vi "Initialize Sourcemeter (Pratap).vi"(5 "Source Value":dbl, 7 "Compliance Limit":dbl, 8 "error in (no error)":errorcluster, 9 "Reset (True)":bool, 10 "Source Function":enum32{"Current", "Voltage"}(ring), 11 "VISA Refnum in":refnum<visa-resource-name>) -> (0 "error out":errorcluster, 2 "Node Out":string, 3 "VISA Refnum out":refnum<visa-resource-name>)   [LabVIEW 2025, in "MySMU.lvlib"]
uses:
  MySMU.lvlib
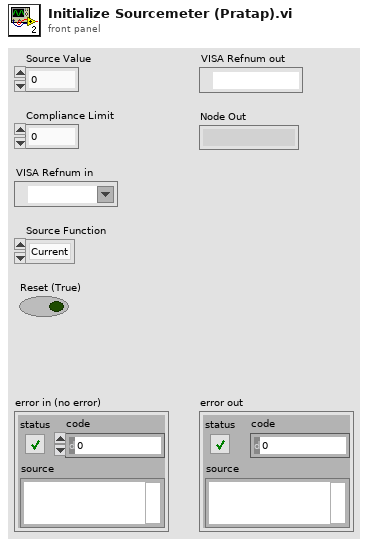
[diagram p1: front panel]
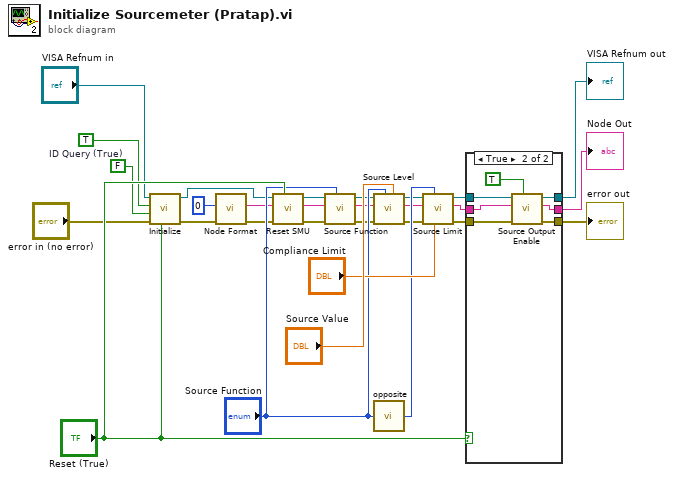
[diagram p0: block diagram]
diagram:
  w3 = TRUE  # ID Query (True)
  n1 = call "Initialize.vi"("Reset (True)"="Reset (True)", "error in (no error)"="error in (no error)", "Error Query (False)"=FALSE, "ID Query (True)"=w3, "VISA resource name"="VISA Refnum in") -> ("error out"=w13:errorcluster, "VISA resource name out"=w5:refnum<visa-resource-name>)  [unwired: 1 in, 4 out]
  n2 = call "Node Format.vi"("error in"=w13, "Node (0-64)"=i8 0) -> ("error out"=w14:errorcluster, "Formatted Node"=w12:string)  [unwired: 8 out]
  n3 = call "Reset SMU.vi"("SMU A (No)"="Reset (True)", "error in (no error)"=w14, "Node In"=w12, "VISA resource name"=w5) -> ("error out"=w6:errorcluster, "Node Out"=w8:string, "VISA resource name out"=w7:refnum<visa-resource-name>)  [unwired: 1 in, 4 out]
  n4 = call "Source Function.vi"("Function (Source)"="Source Function", "error in (no error)"=w6, "Node In"=w8, "VISA resource name"=w7) -> ("error out"=w11:errorcluster, "Node Out"=w9:string, "VISA resource name out"=w10:refnum<visa-resource-name>)  [unwired: 1 in, 4 out]
  n5 = call "Source Level.vi"("Level (0.000)"="Source Value", "Function (Current)"="Source Function", "error in (no error)"=w11, "Node In"=w9, "VISA resource name"=w10) -> ("error out"=w16:errorcluster, "Node Out"=w17:string, "VISA resource name out"=w18:refnum<visa-resource-name>)  [unwired: 1 in, 3 out]
  n6 = call "opposite.vi"("x 2"="Source Function") -> ("x"=w20:enum32{"Current", "Voltage"})
  n7 = call "Source Limit.vi"("Limit (0.000)"="Compliance Limit", "Function (Current)"=w20, "error in (no error)"=w16, "Node In"=w17, "VISA resource name"=w18) -> ("error out"=w25:errorcluster, "Node Out"=w24:string, "VISA resource name out"=w23:refnum<visa-resource-name>)  [unwired: 1 in, 3 out]
  n8 = case shown="True" "Reset (True)" {
    tunnel: w23 -> [w32 w39]
    tunnel: w24 -> [w31 w38]
    tunnel: w25 -> [w30 w37]
    tunnel: [w32 w36] -> w26
    tunnel: [w31 w35] -> w27
    tunnel: [w30 w34] -> w28
    frame False {
    }
    frame True {
      n9 = call "Source Output Enable.vi"("Output (Off)"=TRUE, "error in (no error)"=w37, "Node In"=w38, "VISA resource name"=w39) -> ("error out"=w34:errorcluster, "Node Out"=w35:string, "VISA resource name out"=w36:refnum<visa-resource-name>)  [unwired: 1 in, 4 out]
    }
  }
  "error out" <- w28
  "Node Out" <- w27
  "VISA Refnum out" <- w26
